vi "String Test.vi"() -> ()   [LabVIEW 2014]
panel:
  out "offset past match":i32
  out "after substring":string
  out "match substring":string
  out "before substring":string
  in  "offset (0)":i32
  in  "regular expression":string
  in  "string":string
  out "output 2":dbl
  out "output 1":string
  out "time stamp":timestamp
  out "F-format string":string
  out "Time Stamp 2":timestamp
  out "Numeric":dbl
  in  "Time Stamp":timestamp
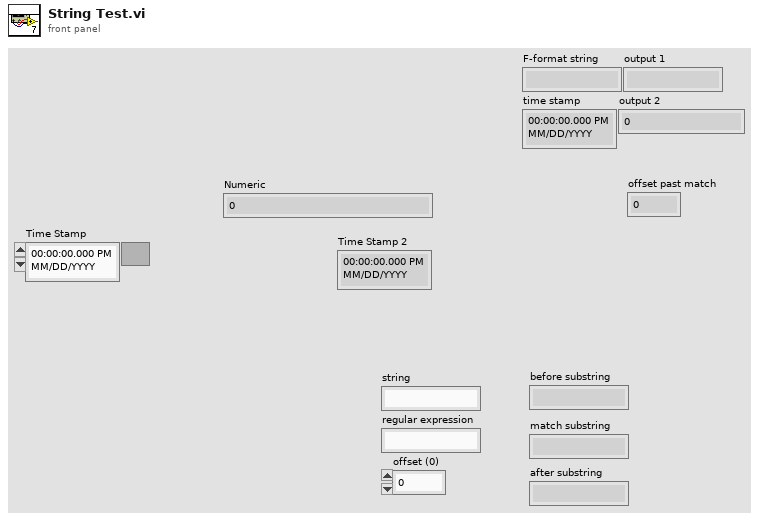
[diagram p1: front panel]
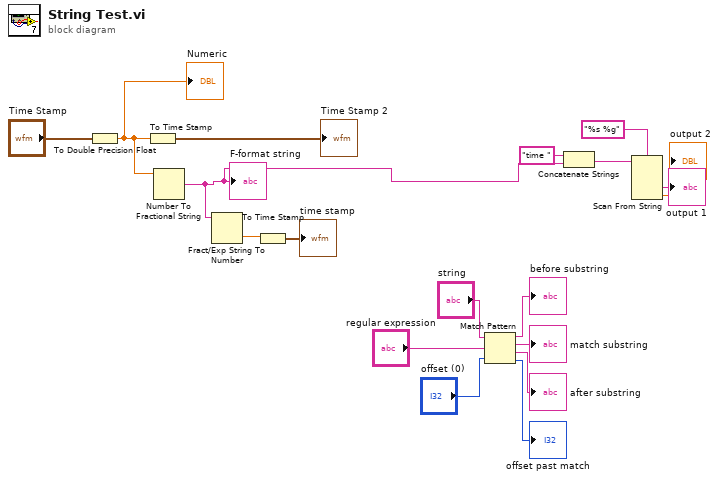
[diagram p0: block diagram]
diagram:
  n1 = To Double Precision Float(number="Time Stamp") -> (double precision float=w16:dbl)
  "Numeric" <- w16
  n2 = To Time Stamp(1:w16) -> (0:→"Time Stamp 2":timestamp)
  n3 = Number To Fractional String(number=w16) -> (F-format string=w13:string)  [unwired: 3 in]
  "F-format string" <- w13
  n4 = Fract/Exp String To Number(string=w13) -> (number=w15:dbl)  [unwired: 3 in, 1 out]
  n5 = To Time Stamp(1:w15) -> (0:→"time stamp":timestamp)
  n6 = Match Pattern(string="string", regular expression="regular expression", offset (0)="offset (0)") -> (before substring=→"before substring":string, match substring=→"match substring":string, after substring=→"after substring":string, offset past match=→"offset past match":i32)
  n7 = Concatenate Strings("time " ("string"), w13) -> (w11:string)
  n8 = Scan From String(format string="%s %g", input string=w11) -> (output 1=→"output 1":string, output 2=→"output 2":dbl)  [unwired: 4 in, 3 out]
